vi "MICSD Get Info.vi"(8 "error in (no error)":errorcluster, 10 "Command":T1(ring), 11 "VISA Resource Name":refnum<visa-resource-name>) -> (0 "error out":errorcluster, 2 "Response":string, 3 "dup VISA Resource Name":refnum<visa-resource-name>)   [LabVIEW 2020]
uses:
  <vilib>/Instr/_visa.llb/VISA Configure Serial Port (Instr).vi
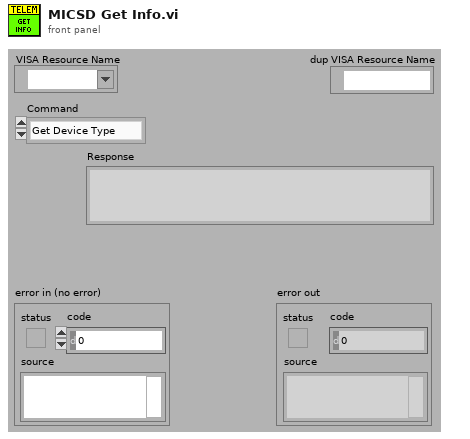
[diagram p1: front panel]
types:
  T1 = enum16{"Get Device Type", "Get Device Name", "Get Device Version", "Get Device Error"}
  T2 = cluster{"Command Token":u8, "Length":u16, "Pack Data":u8[]}
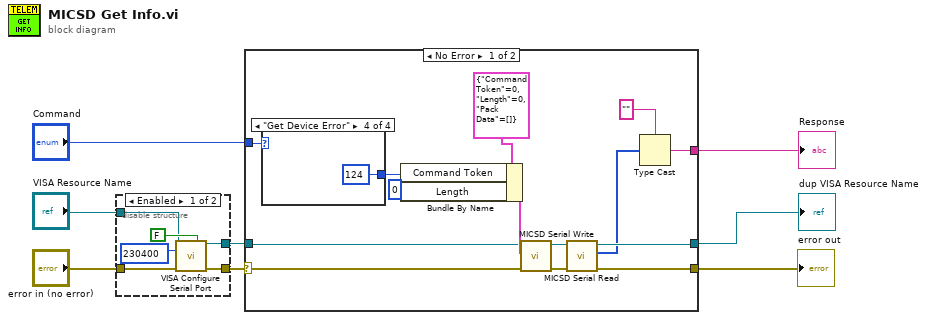
[diagram p0: block diagram]
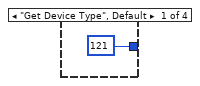
[diagram p3: hidden frame]
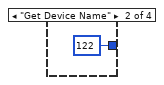
[diagram p4: hidden frame]
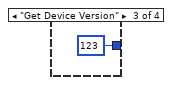
[diagram p5: hidden frame]
diagram:
  n1 = disable-structure shown="Enabled" {
    disable-tunnel: [w12 w15] -> w7
    disable-tunnel: "error in (no error)" -> [w11 w15]
    disable-tunnel: "VISA Resource Name" -> [w10 w16]
    disable-tunnel: [w9 w16] -> w4
    frame Enabled {
      n2 = call-poly "VISA Configure Serial Port"("VISA resource name"=w10, "Enable Termination\nChar (T)"=FALSE ("Enable Termination\nChar (T)"), "baud rate (9600)"=u32 230400, "error in (no error)"=w11) -> ("VISA resource name out"=w9:refnum<visa-resource-name>, "error out"=w12:errorcluster)  [unwired: 10 in]
    }
    frame Disabled {
    }
  }
  n3 = case shown="No Error" w7 {
    selector: w7 -> [w28 w37]
    tunnel: [w25 w37] -> w1
    tunnel: w4 -> [w27 w36]
    tunnel: [w26 w36] -> w8
    tunnel: [w22 "" ("type")] -> w3
    tunnel: "Command" -> [w21 _]
    frame No Error {
      n4 = case shown="\"Get Device Error\"" w21 {
        tunnel: [u16 121 ("Length") u16 122 ("Length") u16 123 ("Length") u16 124 ("Length")] -> w20
        frame "Get Device Type", Default {
        }
        frame "Get Device Name" {
        }
        frame "Get Device Version" {
        }
        frame "Get Device Error" {
        }
      }
      n5 = Bundle By Name(cluster=T2 {"Command Token"=0, "Length"=0, "Pack Data"=[]} ("Write Data"), "Command Token"=w20, "Length"=u16 0) -> (w30:T2)
      n6 = call "MICSD Serial Write.vi"("error in (no error)"=w28, "Write Data"=w30, "VISA Resource Name"=w27) -> ("error out"=w17:errorcluster, "DUP Visa Resource Name"=w18:refnum<visa-resource-name>)  [unwired: 7 in]
      n7 = call "MICSD Serial Read.vi"("error in (no error)"=w17, "VISA Resource Name"=w18) -> ("error out"=w25:errorcluster, "Read Data"=w24:u8[], "DUP Visa Resource Name"=w26:refnum<visa-resource-name>)  [unwired: 7 in]
      n8 = Type Cast(type="", x=w24) -> (*(type *) &x=w22:string)
    }
    frame Error {
    }
  }
  "dup VISA Resource Name" <- w8
  "error out" <- w1
  "Response" <- w3
